vi "LTVDiffDriveCtrl_Pack_Model_Params.vi"(5 "LTV_DiffDriveCtrl_Control":T2={"Max left vel ctrl effort V"=12.0, "Desired Heading Ctrl Tol Rad"=0.06, "Desired Y Pos Meas Tol M"=0.125, "Desired X Pos Ctrl Tol M"=0.125, "Desired Left Vel Ctrl Tol M/S"=0.1, "Desired Right Vel Ctrl Tol M/S"=0.1, "Max right vel ctrl effort V"=12.0} {"Max right vel ctrl effort V" format="%#_13g"; "Desired Right Vel Ctrl Tol M/S" format="%#_13g"; "Desired Left Vel Ctrl Tol M/S" format="%#_13g"; "Desired X Pos Ctrl Tol M" format="%#_13g"; "Desired Y Pos Meas Tol M" format="%#_13g"; "Desired Heading Ctrl Tol Rad" format="%#_13g"; "Max left vel ctrl effort V" format="%#_13g"}, 7 "LTV_DiffDriveCtrl_Tolerance":T1={"Max Heading Tolerance Rad"=0.2, "Max X Tolerance M"=0.0625, "Max Y Tolerance M"=0.125, "Max Left Vel Tol M/S"=0.2, "Max Right Vel Tol M/S"=0.2} {"Max Right Vel Tol M/S" format="%#_13g"; "Max Left Vel Tol M/S" format="%#_13g"; "Max Y Tolerance M" format="%#_13g"; "Max X Tolerance M" format="%#_13g"; "Max Heading Tolerance Rad" format="%#_13g"}, 8 "dT Sec":dbl=0.02, 10 "Track Width":dbl, 11 "Diff_Drive_Linear_System":T3) -> (3 "LTV_DiffDriveCtrl_Model":T5={"Track Width"=0.0, "Diff_Drive_Linear_System"={"m_A"=[], "m_B"=[], "m_C"=[], "m_D"=[], "States"=0, "Inputs"=0, "Outputs"=0}, "LTV_DiffDriveCtrl_Control"={"Max left vel ctrl effort V"=12.0, "Desired Heading Ctrl Tol Rad"=0.06, "Desired Y Pos Meas Tol M"=0.125, "Desired X Pos Ctrl Tol M"=0.125, "Desired Left Vel Ctrl Tol M/S"=0.1, "Desired Right Vel Ctrl Tol M/S"=0.1, "Max right vel ctrl effort V"=12.0}, "LTV_DiffDriveCtrl_Tolerance"={"Max Heading Tolerance Rad"=0.2, "Max X Tolerance M"=0.0625, "Max Y Tolerance M"=0.125, "Max Left Vel Tol M/S"=0.2, "Max Right Vel Tol M/S"=0.2}, "dT Sec"=0.2} {"LTV_DiffDriveCtrl_Tolerance"."Max Right Vel Tol M/S" format="%#_13g"; "LTV_DiffDriveCtrl_Tolerance"."Max Left Vel Tol M/S" format="%#_13g"; "LTV_DiffDriveCtrl_Tolerance"."Max Y Tolerance M" format="%#_13g"; "LTV_DiffDriveCtrl_Tolerance"."Max X Tolerance M" format="%#_13g"; "LTV_DiffDriveCtrl_Tolerance"."Max Heading Tolerance Rad" format="%#_13g"; "LTV_DiffDriveCtrl_Control"."Max right vel ctrl effort V" format="%#_13g"; "LTV_DiffDriveCtrl_Control"."Desired Right Vel Ctrl Tol M/S" format="%#_13g"; "LTV_DiffDriveCtrl_Control"."Desired Left Vel Ctrl Tol M/S" format="%#_13g"; "LTV_DiffDriveCtrl_Control"."Desired X Pos Ctrl Tol M" format="%#_13g"; "LTV_DiffDriveCtrl_Control"."Desired Y Pos Meas Tol M" format="%#_13g"; "LTV_DiffDriveCtrl_Control"."Desired Heading Ctrl Tol Rad" format="%#_13g"; "LTV_DiffDriveCtrl_Control"."Max left vel ctrl effort V" format="%#_13g"; "Track Width" format="%#_13g"})   [LabVIEW 2019, in "Trajectory_Library.lvlib"]
doc: "Pack model, control, and tolerance values for LTV Diff Drive control execute function:\n\nInputs:\n - LTV Diff Drve Ctrl -- cluster -- Packed control parameters\n - LTV Diff Drive Tol -- cluster -- Packed tolerance parameters\n - Diff Drive Linear System -- Linear system -- Diff Drive linear system\n - Track Width -- double -- Track width (meters)\n - dT Sec -- double -- Update time (Default 0.02)\n\nOutputs:\n - LTVDiffDrveCtrlModel -- cluster -- Packed model, control, tolerance values"
uses:
  Trajectory_Library.lvlib
  TypeDef/LTV_DIFF_DRIVE_CTRL_MODEL_PARAMS.CTL
  TypeDef/LINEAR_SYSTEM.ctl
  <vilib>/Analysis/Matrix/Datatypes/RealMatrix.ctl
  TypeDef/LTV_DIFF_DRIVE_CTRL_CONTROL_PARAMS.CTL
  TypeDef/LTV_DIFF_DRIVE_CTRL_TOLERANCE.CTL
  <vilib>/Analysis/Matrix/NI_Matrix.lvlib
panel:
  # "<States,States>"
  # "<States,Inputs>"
  # "<Outputs,States>"
  # "<Outputs,Inputs>"
  # "<States,States>"
  # "<States,Inputs>"
  # "<Outputs,States>"
  # "<Outputs,Inputs>"
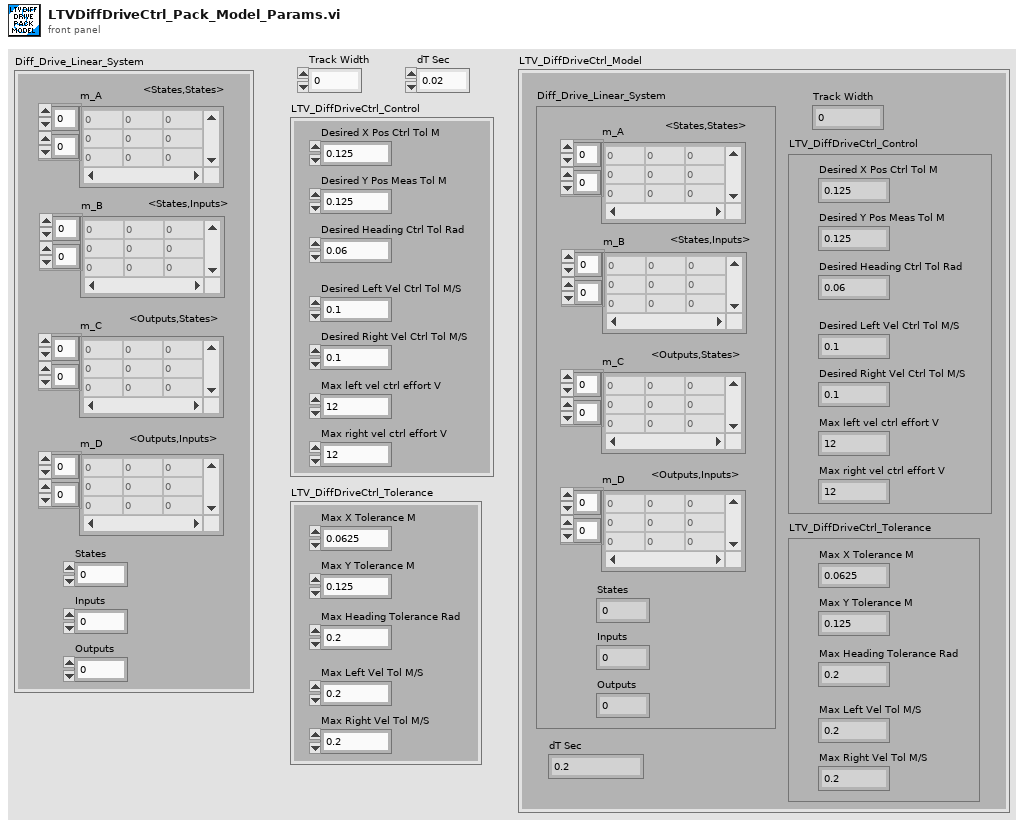
[diagram p1: front panel]
types:
  T1 = typedef "Trajectory_Library.lvlib/LTV_DIFF_DRIVE_CTRL_TOLERANCE.CTL" = cluster{"Max Heading Tolerance Rad":dbl, "Max X Tolerance M":dbl, "Max Y Tolerance M":dbl, "Max Left Vel Tol M/S":dbl, "Max Right Vel Tol M/S":dbl}
  T2 = typedef "Trajectory_Library.lvlib/LTV_DIFF_DRIVE_CTRL_CONTROL_PARAMS.CTL" = cluster{"Max left vel ctrl effort V":dbl, "Desired Heading Ctrl Tol Rad":dbl, "Desired Y Pos Meas Tol M":dbl, "Desired X Pos Ctrl Tol M":dbl, "Desired Left Vel Ctrl Tol M/S":dbl, "Desired Right Vel Ctrl Tol M/S":dbl, "Max right vel ctrl effort V":dbl}
  T3 = typedef "Trajectory_Library.lvlib/LINEAR_SYSTEM.ctl" = cluster{"m_A":T4, "m_B":T4, "m_C":T4, "m_D":T4, "States":i32, "Inputs":i32, "Outputs":i32}
  T4 = typedef "NI_Matrix.lvlib/RealMatrix.ctl" = dbl[][]
  T5 = typedef "Trajectory_Library.lvlib/LTV_DIFF_DRIVE_CTRL_MODEL_PARAMS.CTL" = cluster{"Track Width":dbl, "Diff_Drive_Linear_System":T3, "LTV_DiffDriveCtrl_Control":T2, "LTV_DiffDriveCtrl_Tolerance":T1, "dT Sec":dbl}
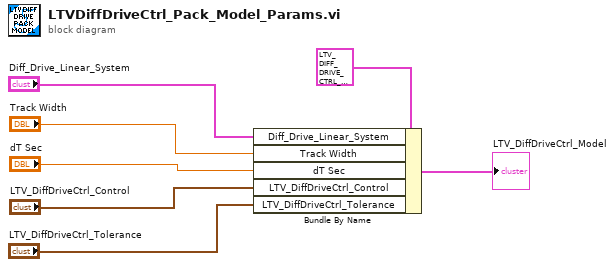
[diagram p0: block diagram]
diagram:
  n1 = Bundle By Name(cluster=T5 {"Track Width"=8.0, "Diff_Drive_Linear_System"={"m_A"=[], "m_B"=[], "m_C"=[], "m_D"=[], "States"=0, "Inputs"=0, "Outputs"=0}, "LTV_DiffDriveCtrl_Control"={"Max left vel ctrl effort V"=12.0, "Desired Heading Ctrl Tol Rad"=0.06, "Desired Y Pos Meas Tol M"=0.125, "Desired X Pos Ctrl Tol M"=0.125, "Desired Left Vel Ctrl Tol M/S"=0.1, "Desired Right Vel Ctrl Tol M/S"=0.1, "Max right vel ctrl effort V"=12.0}, "LTV_DiffDriveCtrl_Tolerance"={"Max Heading Tolerance Rad"=0.2, "Max X Tolerance M"=0.0625, "Max Y Tolerance M"=0.125, "Max Left Vel Tol M/S"=0.2, "Max Right Vel Tol M/S"=0.2}, "dT Sec"=0.2} ("SngJntArmSim_Simulation _Params"), "Diff_Drive_Linear_System"="Diff_Drive_Linear_System", "Track Width"="Track Width", "dT Sec"="dT Sec", "LTV_DiffDriveCtrl_Control"="LTV_DiffDriveCtrl_Control", "LTV_DiffDriveCtrl_Tolerance"="LTV_DiffDriveCtrl_Tolerance") -> (→"LTV_DiffDriveCtrl_Model":T5)
